vi "add.vi"(8 "error in (no error)":errorcluster, 9 "vi refnum":refnum<vi>, 10 "name":string, 11 "window in":refnum<class "rywindow.lvclass">) -> (0 "error out":errorcluster, 3 "window out":refnum<class "rywindow.lvclass">)   [LabVIEW 2017, in "rywindow.lvclass"]
uses:
  rywindow.lvclass
  rywindow.lvclass/rywindow.ctl
  thread.ctl
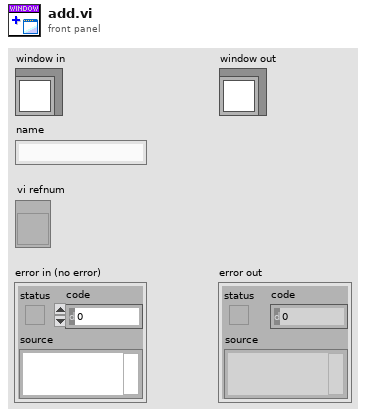
[diagram p1: front panel]
types:
  T1 = typedef "rywindow.lvclass/thread.ctl" = cluster{"name":string, "vi":refnum<vi>}
  T2 = typedef "rywindow.lvclass/data.ctl" = cluster{"threads":T1[], "MinSize":cluster{"Width":u32, "Height":u32}, "font":T3, "active":i32}
  T3 = typedef "LVFontTypeDef.ctl" = cluster{"Font Name":string, "Size":u16, "Bold":bool, "Italic":bool, "Underline":bool, "Strikeout":bool, "Color":u32}
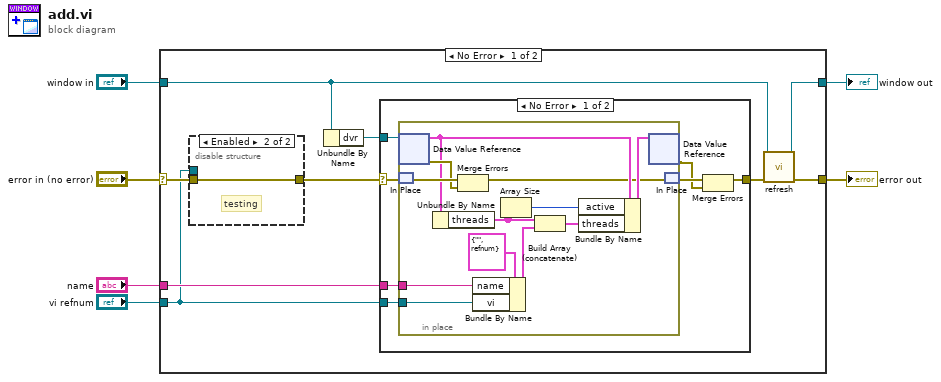
[diagram p0: block diagram]
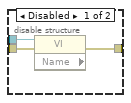
[diagram p2: hidden frame]
diagram:
  n1 = case shown="No Error" "error in (no error)" {
    selector: "error in (no error)" -> [w14 w41]
    tunnel: [w13 w41] -> w5
    tunnel: [w10 w40] -> w3
    tunnel: "window in" -> [w11 w40]
    tunnel: "name" -> [w9 _]
    tunnel: "vi refnum" -> [w7 _]
    frame No Error {
      n2 = disable-structure shown="Enabled" {
        disable-tunnel: w14 -> [w18 w19]
        disable-tunnel: [w17 w19] -> w8
        disable-tunnel: w7 -> [w16 _]
        frame Disabled {
          n3 = property class="VI" props=["Name"](reference=w16, error in=w18) -> (error out=w17:errorcluster)  [unwired: 2 out]
        }
        frame Enabled {
          # "testing"
        }
      }
      n4 = Unbundle By Name(w11) -> ("dvr"=w15:refnum<data-value>)
      n5 = case shown="No Error" w8 {
        selector: w8 -> [w21 w39]
        tunnel: w15 -> [w26 _]
        tunnel: [w23 w39] -> w12
        tunnel: w9 -> [w22 _]
        tunnel: w7 -> [w20 _]
        frame No Error {
          n6 = in-place {
            in-place-border: w22 -> [w32]
            in-place-border: w20 -> [w31]
            n7 = in-place-dvr #1(w26) -> (w36:T2, w37:errorcluster)
            n8 = in-place-match #2(w21) -> (w38:errorcluster)
            n9 = Unbundle By Name(w36) -> ("threads"=w27:T1[])
            n10 = Merge Errors(w38, w37) -> (w34:errorcluster)
            n11 = Bundle By Name(cluster=T1 {"name"="", "vi"=refnum} ("thread"), "name"=w32, "vi"=w31) -> (w30:T1)
            n12 = Array Size(array=w27) -> (size(s)=w28:i32)
            n13 = Build Array (concatenate)(w27, w30) -> (w29:T1[])
            n14 = Bundle By Name(cluster=w36, "active"=w28, "threads"=w29) -> (w35:T2)
            n15 = in-place-dvr #1(w35) -> (w24:errorcluster)  [unwired: 1 out]
            n16 = in-place-match #2(w34) -> (w25:errorcluster)
          }
          n17 = Merge Errors(w25, w24) -> (w23:errorcluster)
        }
        frame Error {
        }
      }
      n18 = call "refresh.vi"("error in (no error)"=w12, "window in"=w11) -> ("error out"=w13:errorcluster, "window out"=w10:refnum<class "rywindow.lvclass">)  [unwired: 8 in]
    }
    frame Error {
    }
  }
  "error out" <- w5
  "window out" <- w3
